vi "Static Ctor.vi"(8 "error in (no error)":errorcluster, 11 "Panel in":refnum<class "Panel.lvclass">) -> (0 "error out":errorcluster, 3 "Panel out":refnum<class "Panel.lvclass">)   [LabVIEW 2020, in "OOPanel.lvlib" / "Panel.lvclass"]
uses:
  Panel.lvclass
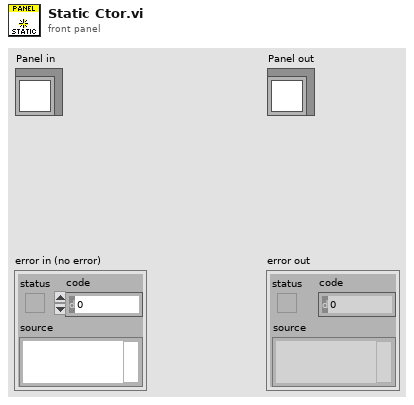
[diagram p1: front panel]
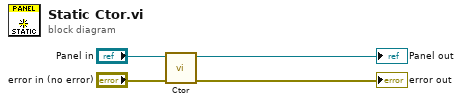
[diagram p0: block diagram]
diagram:
  n1 = call-dynamic "Ctor.vi"("error in (no error)"="error in (no error)", "Panel in"="Panel in") -> ("error out"=→"error out":errorcluster, "Panel out"=→"Panel out":refnum<class "Panel.lvclass">)  [unwired: 8 in]
